vi "Panel Manager Description.vi"(5 "Description":string, 7 "Description Title":string, 8 "error in (no error)":errorcluster, 9 "Stop Event":refnum<user-event>, 10 "Panel":refnum<class "Panel.lvclass">) -> (0 "error out":errorcluster)   [LabVIEW 2020]
doc: "Shows a description for the panel manager being shown off.\n----\nCopyright: MGI 2017\nAuthor: Derek Trepanier"
uses:
  <vilib>/MGI/Panel Manager/Panel/Panel/Panel.lvclass
panel:
  out "MGI Panel Manager":string="The MGI Panel Manager is a framework to help developers quickly implement complex user interfaces by providing an extendable way to define how to show the a VI's front panel. Panels can be their own window, inserted into a subpanel or any number of other display types. The complicated UI code can be written once, then reused across many projects."
  out "Description Display":string caption="Changing Panels"
  # "Visit http://www.mooregoodideas.com for more info."
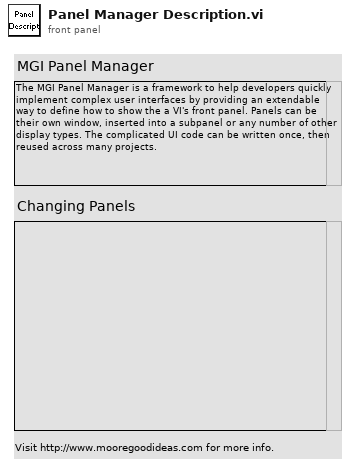
[diagram p1: front panel]
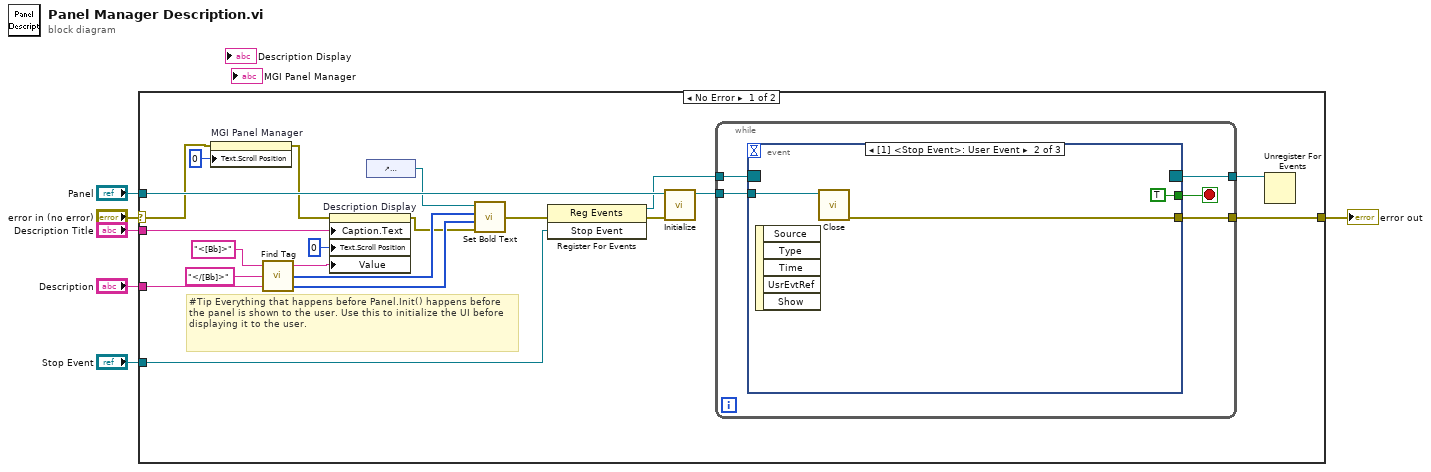
[diagram p0: block diagram]
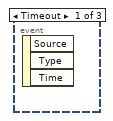
[diagram p2: hidden frame]
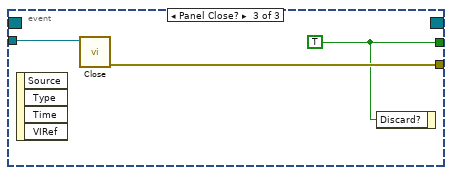
[diagram p3: hidden frame]
diagram:
  n1 = case shown="No Error" "error in (no error)" {
    selector: "error in (no error)" -> [w9 w39]
    tunnel: "Description Title" -> [w27 _]
    tunnel: "Stop Event" -> [w26 _]
    tunnel: [w22 w39] -> w3
    tunnel: "Panel" -> [w21 _]
    tunnel: "Description" -> [w20 _]
    frame No Error {
      # "#Tip Everything that happens before Panel.Init() happens before the panel is shown to the user. Use this to initialize the UI before displaying it to the user."
      n2 = property on="MGI Panel Manager" class="Str"(error in=w9, "Text.Scroll Position"=u32 0) -> (error out=w8:errorcluster)  [unwired: 1 in, 1 out]
      n3 = call <vilib>:"Find Tag.vi"("string"=w20, "close tag"="</[Bb]>" ("don't translate!"), "open tag"="<[Bb]>" ("don't translate!")) -> ("Length"=w18:i32[], "Start"=w19:i32[], "string out"=w12:string)
      n4 = property on="Description Display" class="Str"(error in=w8, "Caption.Text"=w27, "Text.Scroll Position"=u32 0, "Value"=w12) -> (error out=w17:errorcluster)  [unwired: 1 in, 1 out]
      n5 = control-ref of="Description Display"() -> (w13:refnum<vi>)
      n6 = call <vilib>:"Set Bold Text.vi"("error in"=w17, "Length"=w18, "Start"=w19, "text"=w13) -> ("error out"=w16:errorcluster)  [unwired: 2 in]
      n7 = register-events(error in=w16, w26) -> (reference out=w7:refnum<event-registration>, error out=w25:errorcluster)  [unwired: 1 in]
      n8 = call <vilib>:"Initialize.vi"("error in (no error)"=w25, "Panel In"=w21) -> ("Panel Out"=w24:refnum<class "Panel.lvclass">)  [unwired: 7 in, 2 out]
      n9 = while {
        tunnel: w24 -> [w32]
        tunnel: w7 -> [w31]
        tunnel: [w29] -> w23
        tunnel: [w28] -> w22
        stop <- w30 stop-if-true
        n10 = event shown="[1] <Stop Event>: User Event" {
          selector: w31 -> [_ _ _]
          dyn-events: [_ _ _] -> w29
          timeout: _ -> [_ _ _]
          tunnel: w32 -> [_ w34 w38]
          tunnel: [_ TRUE w36] -> w30
          tunnel: [_ w33 w37] -> w28
          event Timeout {
            n11 = event-data() -> ()  [unwired: 1 in, 3 out]
          }
          event User Event {
            n12 = event-data() -> ()  [unwired: 1 in, 5 out]
            n13 = call-dynamic "Close.vi"("Panel In"=w34) -> ("Error Out"=w33:errorcluster)  [unwired: 10 in]
          }
          event Panel Close? {
            w36 = TRUE
            n14 = event-data() -> ()  [unwired: 1 in, 4 out]
            n15 = call-dynamic "Close.vi"("Panel In"=w38) -> ("Error Out"=w37:errorcluster)  [unwired: 10 in]
            n16 = event-data("Discard?"=w36) -> ()  [unwired: 1 in, 1 out]
          }
        }
      }
      n17 = Unregister For Events(event registration refnum=w23) -> ()  [unwired: 1 in, 1 out]
    }
    frame Error {
    }
  }
  "error out" <- w3
